vi "Get Technology.vi"(8 "error in (no error)":errorcluster, 11 "niDTS GNSS DUT in":refnum<class "niDTS GNSS Dut.lvclass">) -> (0 "error out":errorcluster, 2 "Technology":string, 3 "niDTS GNSS DUT out":refnum<class "niDTS GNSS Dut.lvclass">)   [LabVIEW 2015, in "niDTS GNSS.lvlib" / "niDTS GNSS Dut.lvclass"]
uses:
  niDTS GNSS Dut.lvclass
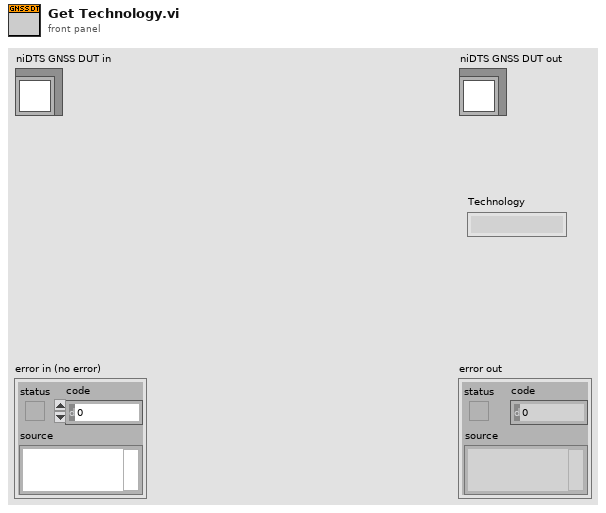
[diagram p1: front panel]
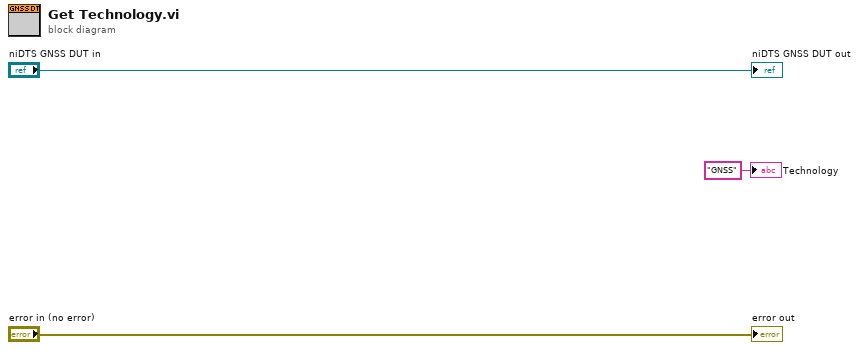
[diagram p0: block diagram]
diagram:
  "error out" <- "error in (no error)"
  "niDTS GNSS DUT out" <- "niDTS GNSS DUT in"
  "Technology" <- "GNSS" ("Technology")
